vi "XNET UDP Socket Write (Text).vi"(5 "remote port":u16, 7 "remote address":string, 8 "error in":errorcluster, 9 "timeout ms (25000)":i32=25000, 10 "data":string, 11 "socket in":refnum<k20>) -> (0 "error out":errorcluster, 3 "socket out":refnum<k20>)   [LabVIEW 2018]
doc: "Writes string data to a UDP network connection."
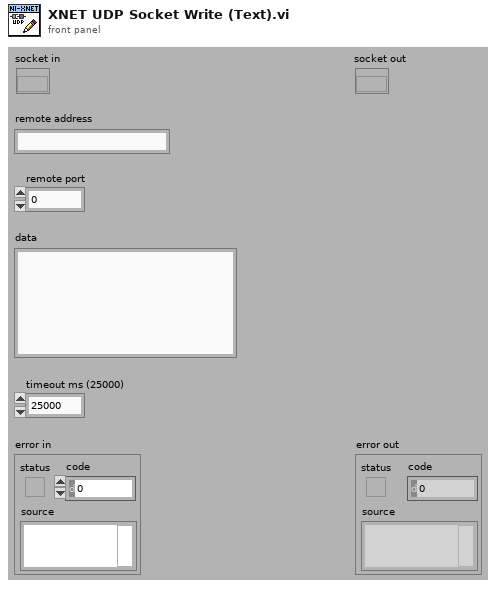
[diagram p1: front panel]
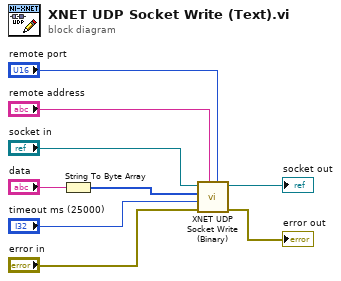
[diagram p0: block diagram]
diagram:
  n1 = String To Byte Array(string="data") -> (unsigned byte array=w5:u8[])
  n2 = call "XNET UDP Socket Write (Binary).vi"("remote port"="remote port", "remote address"="remote address", "error in"="error in", "timeout ms (25000)"="timeout ms (25000)", "data"=w5, "socket in"="socket in") -> ("error out"=→"error out":errorcluster, "socket out"=→"socket out":refnum<k20>)  [unwired: 4 in]
